vi "test_libssh2_session_read_timeout.vi"() -> ()   [LabVIEW 2017, in "unit_tests.lvlib"]
uses:
  unit_tests.lvlib
  libssh2/libssh2_init_default.vi
  libssh2/libssh2_session_init_ex.vi
  libssh2/libssh2.lvlib
  <vilib>/PNR/Transparent Assertions/Transparent Assertions/Transparent Assertions.lvlib
panel:
  out "error out":errorcluster
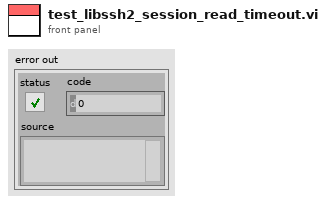
[diagram p1: front panel]
types:
  T1 = typedef "libssh2.lvlib/Session Refnum.ctl" = refnum<k1>
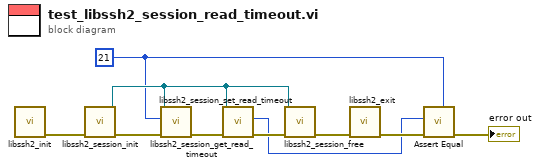
[diagram p0: block diagram]
diagram:
  w1 = 21 ("timeout in ms (0 = indefinite)")
  n1 = call-poly "libssh2_init.vi"() -> ("error out"=w9:errorcluster)  [unwired: 11 in]
  n2 = call "libssh2_session_init.vi"("error in (no error)"=w9) -> ("error out"=w2:errorcluster, "session"=w4:T1)  [unwired: 9 in]
  n3 = call "libssh2_session_set_read_timeout.vi"("error in (no error)"=w2, "read timeout in seconds (0 = default)"=w1, "session"=w4) -> ("error out"=w7:errorcluster)  [unwired: 8 in]
  n4 = call "libssh2_session_get_read_timeout.vi"("error in (no error)"=w7, "session"=w4) -> ("error out"=w5:errorcluster, "read timeout in seconds"=w3:i32)  [unwired: 8 in]
  n5 = call "libssh2_session_free.vi"("error in (no error)"=w5, "session"=w4) -> ("error out"=w8:errorcluster)  [unwired: 9 in]
  n6 = call "libssh2_exit.vi"("error in (no error)"=w8) -> ("error out"=w6:errorcluster)  [unwired: 10 in]
  n7 = call <vilib>:"Assert Equal.vi"("Expected"=w1, "error in (no error)"=w6, "Actual"=w3) -> ("error out"=→"error out":errorcluster)  [unwired: 8 in]
